vi "Tank Drive Immediate.vi"(4 "Right Joystick Y-Axis":dbl, 6 "Right Joystick X-Axis":dbl, 7 "Description":string, 8 "Command Info In":T1, 9 "Deadband":dbl, 10 "Left Joystick Y-Axis":dbl, 11 "Left Joystick X-Axis":dbl) -> (0 "Command Info Out":T1)   [LabVIEW 2020]
doc: "This VI compares the input value to the deadband and optionally notifies the subsystem of the new setpoint."
uses:
  <vilib>/Rock Robotics/WPI/Framework/Command Status Info.ctl
  <vilib>/Rock Robotics/WPI/Framework/Completion Status.ctl
  <vilib>/Rock Robotics/WPI/Framework/Completion Notifier.ctl
  Implementation/Drive Setpoints.ctl
  Implementation/Drive Operations.ctl
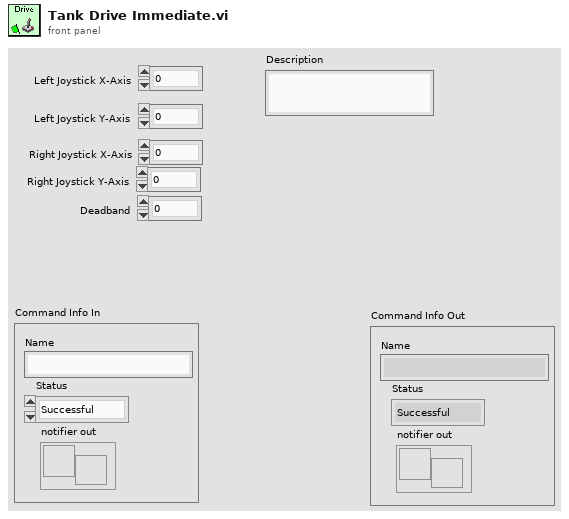
[diagram p1: front panel]
types:
  T1 = typedef "Command Status Info.ctl" = cluster{"Name":string, "Status":T2, "notifier out":T3}
  T2 = typedef "Completion Status.ctl" = enum16{"Successful", "Aborted", "Incomplete"}
  T3 = typedef "Completion Notifier.ctl" = refnum<notifier>
  T4 = typedef "Drive Setpoints.ctl" = cluster{"Operation":T5, "Left Joystick X-Axis":dbl, "Left Joystick Y-Axis":dbl, "Duration":dbl, "Right Joystick Y-Axis":dbl, "Right Joystick X-Axis":dbl}
  T5 = typedef "Drive Operations.ctl" = enum16{"Reserve", "Read Current", "Rocket Drive Immediate", "Tank Drive Immediate", "Drive for Time", "Drive for Distance"}
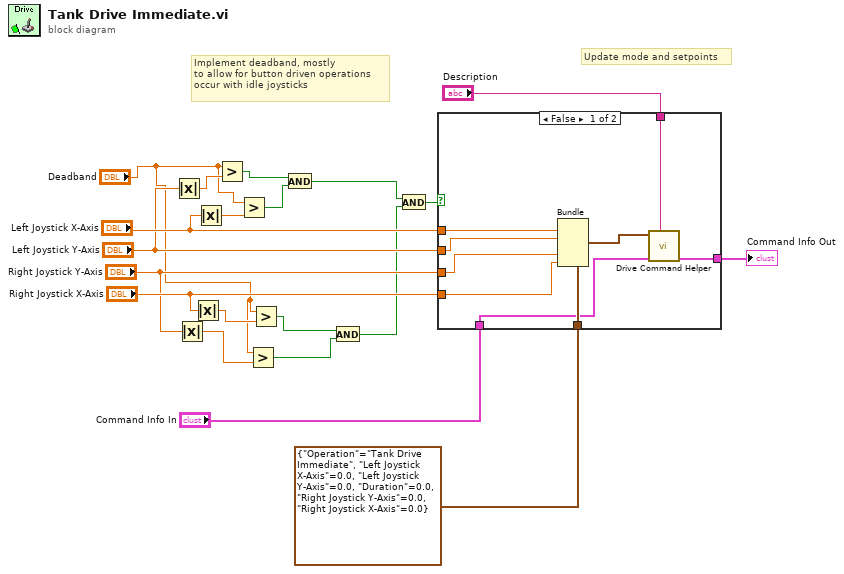
[diagram p0: block diagram]
diagram:
  # "Implement deadband, mostly\nto allow for button driven operations\noccur with idle joysticks"
  # "Update mode and setpoints"
  n1 = Absolute Value(x="Left Joystick Y-Axis") -> (abs(x)=w12:dbl)
  n2 = Absolute Value(x="Right Joystick Y-Axis") -> (abs(x)=w9:dbl)
  n3 = Absolute Value(x="Right Joystick X-Axis") -> (abs(x)=w10:dbl)
  n4 = Absolute Value(x="Left Joystick X-Axis") -> (abs(x)=w11:dbl)
  n5 = Greater?(x="Deadband", y=w12) -> (0:w5:bool)
  n6 = Greater?(x="Deadband", y=w11) -> (0:w4:bool)
  n7 = Greater?(x="Deadband", y=w9) -> (0:w6:bool)
  n8 = Greater?(x="Deadband", y=w10) -> (0:w7:bool)
  n9 = And(x=w5, y=w4) -> (x .and. y?=w3:bool)
  n10 = And(x=w7, y=w6) -> (x .and. y?=w2:bool)
  n11 = And(x=w3, y=w2) -> (x .and. y?=w1:bool)
  n12 = case shown="False" w1 {
    tunnel: T4 {"Operation"=enum."Tank Drive Immediate", "Left Joystick X-Axis"=0.0, "Left Joystick Y-Axis"=0.0, "Duration"=0.0, "Right Joystick Y-Axis"=0.0, "Right Joystick X-Axis"=0.0} ("SubSystem Data") -> [w29 _]
    tunnel: [w28 w30] -> w20
    tunnel: "Command Info In" -> [w25 w30]
    tunnel: "Description" -> [w26 _]
    tunnel: "Left Joystick X-Axis" -> [w24 _]
    tunnel: "Left Joystick Y-Axis" -> [w23 _]
    tunnel: "Right Joystick Y-Axis" -> [w22 _]
    tunnel: "Right Joystick X-Axis" -> [w21 _]
    frame False {
      n13 = Bundle(cluster=w29, "Left Joystick X-Axis"=w24, "Left Joystick Y-Axis"=w23, "Right Joystick Y-Axis"=w22, "Right Joystick X-Axis"=w21) -> (w27:T4)  [unwired: 2 in]
      n14 = call "Drive Command Helper.vi"("Description"=w26, "Command Info In"=w25, "SubSystem Data"=w27) -> ("Command Info Out"=w28:T1)  [unwired: 6 in, 2 out]
    }
    frame True {
    }
  }
  "Command Info Out" <- w20
